vi "Generate Random String.vi"(1 "String Length (Default = 10)":u32=10, 2 "ASCII Character Type":T1) -> (0 "Random String":string)   [LabVIEW 2022 SP3]
doc: "Generates a random string of a given character type and given length.\n\nThis VI can be useful to generate dummy file or folder names, usernames, etc.\n\nPerformance: This VI is inlined to increase performance"
uses:
  ASCII Character Type.ctl
  <vilib>/numeric/Random Number (Range).vi
  <vilib>/numeric/Random Number (Range) U64.vi
  <vilib>/numeric/sub_Random U32.vi
panel:
  # "Development\ncontrols/indicators useful for development and testing, but which are not outputs of the VI"
  # "Input\nInputs to the VI"
  # "Output\nOutputs of the VI"
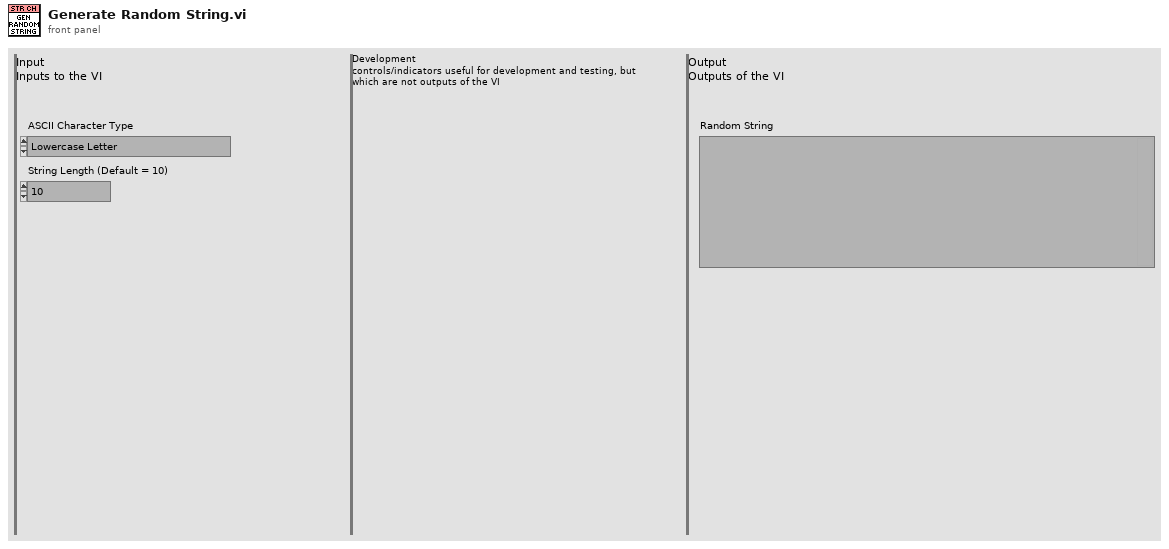
[diagram p1: front panel]
types:
  T1 = typedef "ASCII Character Type.ctl" = enum16{"Lowercase Letter", "Uppercase Letter", "Digit", "Alphanumeric", "Printable Character", "Any ASCII Character [0x00 to 0xFF]"}
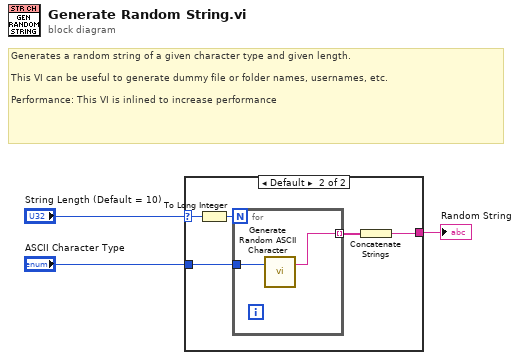
[diagram p0: block diagram]
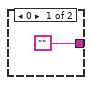
[diagram p2: hidden frame]
diagram:
  # "Generates a random string of a given character type and given length.\n\nThis VI can be useful to generate dummy file or folder names, usernames, etc.\n\nPerformance: This VI is inlined to increase performance"
  n1 = case shown="Default" "String Length (Default = 10)" {
    selector: "String Length (Default = 10)" -> [_ w9]
    tunnel: ["" w7] -> w2
    tunnel: "ASCII Character Type" -> [_ w6]
    frame 0 {
    }
    frame Default {
      n2 = To Long Integer(number=w9) -> (32bit integer=w5:i32)
      n3 = for {
        N: w5 -> [_]
        tunnel: [w11] -> w8 mode=indexing
        tunnel: w6 -> [w10]
        n4 = call "Generate Random ASCII Character.vi"("ASCII Character Type"=w10) -> ("Random ASCII Character"=w11:string)  [unwired: 1 in, 1 out]
      }
      n5 = Concatenate Strings(w8) -> (w7:string)
    }
  }
  "Random String" <- w2
